vi "BCU参数读取-Auto.vi"(8 "CAN端口":u16(ring), 9 "设备索引号":u16(ring), 10 "CAN卡类型":u32(ring)=21, 11 "Myindex":dbl=1.0) -> (3 "成功":bool)   [LabVIEW 2013] (continued)
                n3273 = property on="最大允许温度" class="DigNum (严格)"("Disabled"=w5002) -> ()  [unwired: 2 in, 2 out]
                n3274 = property on="最小允许温度" class="DigNum (严格)"("Disabled"=w5002) -> ()  [unwired: 2 in, 2 out]
                n3275 = property on="最大允许充电电流" class="DigNum (严格)"("Disabled"=w5002) -> ()  [unwired: 2 in, 2 out]
                n3276 = property on="最小允许充电电流" class="DigNum (严格)"("Disabled"=w5002) -> ()  [unwired: 2 in, 2 out]
                n3277 = property on="最小允许单体电压" class="DigNum (严格)"("Disabled"=w5002) -> ()  [unwired: 2 in, 2 out]
                n3278 = property on="电流步长" class="DigNum (严格)"("Disabled"=w5002) -> ()  [unwired: 2 in, 2 out]
                n3279 = property on="SOC" class="DigNum (严格)"("Disabled"=w5002) -> ()  [unwired: 2 in, 2 out]
                n3280 = property on="充电总安时" class="DigNum (严格)"("Disabled"=w5002) -> ()  [unwired: 2 in, 2 out]
                n3281 = property on="放电总安时" class="DigNum (严格)"("Disabled"=w5002) -> ()  [unwired: 2 in, 2 out]
                n3282 = property on="放空次数" class="DigNum (严格)"("DisabledEnum"=w4994) -> ()  [unwired: 2 in, 2 out]
                n3283 = property on="充满次数" class="DigNum (严格)"("DisabledEnum"=w4994) -> ()  [unwired: 2 in, 2 out]
                n3284 = property on="充电次数" class="DigNum (严格)"("DisabledEnum"=w4994) -> ()  [unwired: 2 in, 2 out]
                n3285 = global read "功能码全局.vi" "24"() -> (w4997:bool[])
                n3286 = global read "功能码全局.vi" "23"() -> (w4998:bool[])
                n3287 = Index Array(array=w4997) -> (element #3=w4995:bool)  [unwired: 8 in, 7 out]
                n3288 = Index Array(array=w4998) -> (element #3=w4996:bool)  [unwired: 8 in, 7 out]
                n3289 = Not(x=w4991) -> (.not. x?=w5003:bool)
              }
              frame "电池包组号" {
                w5008 = 2
                w5007 = 2
                w5017 = 2
                w5009 = 2
                w5018 = 2
                w5005 = FALSE ("1 6")
                n3290 = property on="串联数" class="DigNum (严格)"("Disabled"=w5018) -> ()  [unwired: 2 in, 2 out]
                n3291 = property on="并联数" class="DigNum (严格)"("Disabled"=w5018) -> ()  [unwired: 2 in, 2 out]
                n3292 = property on="电池厂家" class="DigNum (严格)"("Disabled"=w5018) -> ()  [unwired: 2 in, 2 out]
                n3293 = property on="电池类型" class="DigNum (严格)"("Disabled"=w5018) -> ()  [unwired: 2 in, 2 out]
                n3294 = property on="额定能量" class="DigNum (严格)"("Disabled"=w5018) -> ()  [unwired: 2 in, 2 out]
                n3295 = property on="额定容量" class="DigNum (严格)"("Disabled"=w5018) -> ()  [unwired: 2 in, 2 out]
                n3296 = property on="实际容量" class="DigNum (严格)"("Disabled"=w5018) -> ()  [unwired: 2 in, 2 out]
                n3297 = Select(t=0, s=w5014, f=1) -> (s? t:f=w5006:i32)
                n3298 = property on="生产日期" class="Str"("DisabledEnum"=w5008) -> ()  [unwired: 2 in, 2 out]
                n3299 = property on="电池包序号" class="DigNum (严格)"("DisabledEnum"=w5008) -> ()  [unwired: 2 in, 2 out]
                n3300 = property on="车牌号" class="Str"("DisabledEnum"=w5008) -> ()  [unwired: 2 in, 2 out]
                n3301 = property on="电池包组号" class="DigNum (严格)"("DisabledEnum"=w5006) -> ()  [unwired: 2 in, 2 out]
                n3302 = property on="电池组信息" class="Clust (严格)"("Disabled"=w5006) -> ()  [unwired: 2 in, 2 out]
                n3303 = property on="产权标识" class="DigNum (严格)"("Disabled"=w5009) -> ()  [unwired: 2 in, 2 out]
                n3304 = property on="应用车型" class="DigNum (严格)"("Disabled"=w5009) -> ()  [unwired: 2 in, 2 out]
                n3305 = property on="额定总压" class="DigNum (严格)"("Disabled"=w5009) -> ()  [unwired: 2 in, 2 out]
                n3306 = property on="放空次数" class="DigNum (严格)"("DisabledEnum"=w5007) -> ()  [unwired: 2 in, 2 out]
                n3307 = property on="充满次数" class="DigNum (严格)"("DisabledEnum"=w5007) -> ()  [unwired: 2 in, 2 out]
                n3308 = property on="充电次数" class="DigNum (严格)"("DisabledEnum"=w5007) -> ()  [unwired: 2 in, 2 out]
                n3309 = property on="最大允许单体电压" class="DigNum (严格)"("Disabled"=w5017) -> ()  [unwired: 2 in, 2 out]
                n3310 = property on="最大允许总电压" class="DigNum (严格)"("Disabled"=w5017) -> ()  [unwired: 2 in, 2 out]
                n3311 = property on="最大允许温度" class="DigNum (严格)"("Disabled"=w5017) -> ()  [unwired: 2 in, 2 out]
                n3312 = property on="最小允许温度" class="DigNum (严格)"("Disabled"=w5017) -> ()  [unwired: 2 in, 2 out]
                n3313 = property on="最大允许充电电流" class="DigNum (严格)"("Disabled"=w5017) -> ()  [unwired: 2 in, 2 out]
                n3314 = property on="最小允许充电电流" class="DigNum (严格)"("Disabled"=w5017) -> ()  [unwired: 2 in, 2 out]
                n3315 = property on="最小允许单体电压" class="DigNum (严格)"("Disabled"=w5017) -> ()  [unwired: 2 in, 2 out]
                n3316 = property on="电流步长" class="DigNum (严格)"("Disabled"=w5017) -> ()  [unwired: 2 in, 2 out]
                n3317 = property on="SOC" class="DigNum (严格)"("Disabled"=w5017) -> ()  [unwired: 2 in, 2 out]
                n3318 = property on="充电总安时" class="DigNum (严格)"("Disabled"=w5017) -> ()  [unwired: 2 in, 2 out]
                n3319 = property on="放电总安时" class="DigNum (严格)"("Disabled"=w5017) -> ()  [unwired: 2 in, 2 out]
                n3320 = global read "功能码全局.vi" "24"() -> (w5012:bool[])
                n3321 = global read "功能码全局.vi" "23"() -> (w5013:bool[])
                n3322 = Index Array(array=w5012) -> (element #3=w5010:bool)  [unwired: 8 in, 7 out]
                n3323 = Index Array(array=w5013) -> (element #3=w5011:bool)  [unwired: 8 in, 7 out]
                n3324 = Not(x=w5005) -> (.not. x?=w5019:bool)
              }
              frame "充放电安时" {
                w5023 = 2
                w5022 = 2
                w5032 = 2
                w5033 = 2
                w5035 = 2
                w5021 = FALSE ("1 6")
                n3325 = property on="串联数" class="DigNum (严格)"("Disabled"=w5035) -> ()  [unwired: 2 in, 2 out]
                n3326 = property on="并联数" class="DigNum (严格)"("Disabled"=w5035) -> ()  [unwired: 2 in, 2 out]
                n3327 = property on="电池厂家" class="DigNum (严格)"("Disabled"=w5035) -> ()  [unwired: 2 in, 2 out]
                n3328 = property on="电池类型" class="DigNum (严格)"("Disabled"=w5035) -> ()  [unwired: 2 in, 2 out]
                n3329 = property on="额定能量" class="DigNum (严格)"("Disabled"=w5035) -> ()  [unwired: 2 in, 2 out]
                n3330 = property on="额定容量" class="DigNum (严格)"("Disabled"=w5035) -> ()  [unwired: 2 in, 2 out]
                n3331 = property on="实际容量" class="DigNum (严格)"("Disabled"=w5035) -> ()  [unwired: 2 in, 2 out]
                n3332 = Select(t=0, s=w5029, f=1) -> (s? t:f=w5028:i32)
                n3333 = property on="生产日期" class="Str"("DisabledEnum"=w5023) -> ()  [unwired: 2 in, 2 out]
                n3334 = property on="电池包序号" class="DigNum (严格)"("DisabledEnum"=w5023) -> ()  [unwired: 2 in, 2 out]
                n3335 = property on="车牌号" class="Str"("DisabledEnum"=w5023) -> ()  [unwired: 2 in, 2 out]
                n3336 = property on="电池包组号" class="DigNum (严格)"("DisabledEnum"=w5023) -> ()  [unwired: 2 in, 2 out]
                n3337 = property on="电池组信息" class="Clust (严格)"("Disabled"=w5028) -> ()  [unwired: 2 in, 2 out]
                n3338 = property on="额定总压" class="DigNum (严格)"("Disabled"=2) -> ()  [unwired: 2 in, 2 out]
                n3339 = property on="产权标识" class="DigNum (严格)"("Disabled"=w5033) -> ()  [unwired: 2 in, 2 out]
                n3340 = property on="应用车型" class="DigNum (严格)"("Disabled"=w5033) -> ()  [unwired: 2 in, 2 out]
                n3341 = property on="放空次数" class="DigNum (严格)"("DisabledEnum"=w5022) -> ()  [unwired: 2 in, 2 out]
                n3342 = property on="充满次数" class="DigNum (严格)"("DisabledEnum"=w5022) -> ()  [unwired: 2 in, 2 out]
                n3343 = property on="充电次数" class="DigNum (严格)"("DisabledEnum"=w5022) -> ()  [unwired: 2 in, 2 out]
                n3344 = property on="最大允许单体电压" class="DigNum (严格)"("Disabled"=w5032) -> ()  [unwired: 2 in, 2 out]
                n3345 = property on="最大允许总电压" class="DigNum (严格)"("Disabled"=w5032) -> ()  [unwired: 2 in, 2 out]
                n3346 = property on="最大允许温度" class="DigNum (严格)"("Disabled"=w5032) -> ()  [unwired: 2 in, 2 out]
                n3347 = property on="最小允许温度" class="DigNum (严格)"("Disabled"=w5032) -> ()  [unwired: 2 in, 2 out]
                n3348 = property on="最大允许充电电流" class="DigNum (严格)"("Disabled"=w5032) -> ()  [unwired: 2 in, 2 out]
                n3349 = property on="最小允许充电电流" class="DigNum (严格)"("Disabled"=w5032) -> ()  [unwired: 2 in, 2 out]
                n3350 = property on="最小允许单体电压" class="DigNum (严格)"("Disabled"=w5032) -> ()  [unwired: 2 in, 2 out]
                n3351 = property on="电流步长" class="DigNum (严格)"("Disabled"=w5032) -> ()  [unwired: 2 in, 2 out]
                n3352 = property on="SOC" class="DigNum (严格)"("Disabled"=w5032) -> ()  [unwired: 2 in, 2 out]
                n3353 = property on="充电总安时" class="DigNum (严格)"("Disabled"=w5028) -> ()  [unwired: 2 in, 2 out]
                n3354 = property on="放电总安时" class="DigNum (严格)"("Disabled"=w5028) -> ()  [unwired: 2 in, 2 out]
                n3355 = Not(x=w5021) -> (.not. x?=w5036:bool)
                n3356 = global read "功能码全局.vi" "24"() -> (w5026:bool[])
                n3357 = global read "功能码全局.vi" "23"() -> (w5027:bool[])
                n3358 = Index Array(array=w5026) -> (element #7=w5024:bool)  [unwired: 8 in, 7 out]
                n3359 = Index Array(array=w5027) -> (element #7=w5025:bool)  [unwired: 8 in, 7 out]
              }
              frame "充电次数" {
                w5041 = 2
                w5050 = 2
                w5051 = 2
                w5042 = 2
                w5052 = 2
                w5038 = FALSE ("1 6")
                n3360 = property on="串联数" class="DigNum (严格)"("Disabled"=w5052) -> ()  [unwired: 2 in, 2 out]
                n3361 = property on="并联数" class="DigNum (严格)"("Disabled"=w5052) -> ()  [unwired: 2 in, 2 out]
                n3362 = property on="电池厂家" class="DigNum (严格)"("Disabled"=w5052) -> ()  [unwired: 2 in, 2 out]
                n3363 = property on="电池类型" class="DigNum (严格)"("Disabled"=w5052) -> ()  [unwired: 2 in, 2 out]
                n3364 = property on="额定能量" class="DigNum (严格)"("Disabled"=w5052) -> ()  [unwired: 2 in, 2 out]
                n3365 = property on="额定容量" class="DigNum (严格)"("Disabled"=w5052) -> ()  [unwired: 2 in, 2 out]
                n3366 = property on="实际容量" class="DigNum (严格)"("Disabled"=w5052) -> ()  [unwired: 2 in, 2 out]
                n3367 = Select(t=0, s=w5047, f=1) -> (s? t:f=w5039:i32)
                n3368 = property on="生产日期" class="Str"("DisabledEnum"=w5041) -> ()  [unwired: 2 in, 2 out]
                n3369 = property on="电池包序号" class="DigNum (严格)"("DisabledEnum"=w5041) -> ()  [unwired: 2 in, 2 out]
                n3370 = property on="车牌号" class="Str"("DisabledEnum"=w5041) -> ()  [unwired: 2 in, 2 out]
                n3371 = property on="电池组信息" class="Clust (严格)"("Disabled"=w5039) -> ()  [unwired: 2 in, 2 out]
                n3372 = property on="电池包组号" class="DigNum (严格)"("DisabledEnum"=w5041) -> ()  [unwired: 2 in, 2 out]
                n3373 = property on="额定总压" class="DigNum (严格)"("Disabled"=w5042) -> ()  [unwired: 2 in, 2 out]
                n3374 = property on="产权标识" class="DigNum (严格)"("Disabled"=w5042) -> ()  [unwired: 2 in, 2 out]
                n3375 = property on="应用车型" class="DigNum (严格)"("Disabled"=w5042) -> ()  [unwired: 2 in, 2 out]
                n3376 = property on="放空次数" class="DigNum (严格)"("DisabledEnum"=w5039) -> (error out=w5040:errorcluster)  [unwired: 2 in, 1 out]
                n3377 = property on="充满次数" class="DigNum (严格)"("DisabledEnum"=w5039) -> ()  [unwired: 2 in, 2 out]
                n3378 = property on="充电次数" class="DigNum (严格)"("DisabledEnum"=w5039) -> ()  [unwired: 2 in, 2 out]
                n3379 = property on="最大允许单体电压" class="DigNum (严格)"("Disabled"=w5051) -> ()  [unwired: 2 in, 2 out]
                n3380 = property on="最大允许总电压" class="DigNum (严格)"("Disabled"=w5051) -> ()  [unwired: 2 in, 2 out]
                n3381 = property on="最大允许温度" class="DigNum (严格)"("Disabled"=w5051) -> ()  [unwired: 2 in, 2 out]
                n3382 = property on="最小允许温度" class="DigNum (严格)"("Disabled"=w5051) -> ()  [unwired: 2 in, 2 out]
                n3383 = property on="最大允许充电电流" class="DigNum (严格)"("Disabled"=w5051) -> ()  [unwired: 2 in, 2 out]
                n3384 = property on="最小允许充电电流" class="DigNum (严格)"(error in=w5040, "Disabled"=w5051) -> ()  [unwired: 1 in, 2 out]
                n3385 = property on="最小允许单体电压" class="DigNum (严格)"("Disabled"=w5051) -> ()  [unwired: 2 in, 2 out]
                n3386 = property on="电流步长" class="DigNum (严格)"("Disabled"=w5051) -> ()  [unwired: 2 in, 2 out]
                n3387 = property on="SOC" class="DigNum (严格)"("Disabled"=w5051) -> ()  [unwired: 2 in, 2 out]
                n3388 = property on="充电总安时" class="DigNum (严格)"("Disabled"=w5050) -> ()  [unwired: 2 in, 2 out]
                n3389 = property on="放电总安时" class="DigNum (严格)"("Disabled"=w5050) -> ()  [unwired: 2 in, 2 out]
                n3390 = Not(x=w5038) -> (.not. x?=w5053:bool)
                n3391 = global read "功能码全局.vi" "24"() -> (w5045:bool[])
                n3392 = global read "功能码全局.vi" "23"() -> (w5046:bool[])
                n3393 = Index Array(array=w5045) -> (element #8=w5044:bool)  [unwired: 8 in, 7 out]
                n3394 = Index Array(array=w5046) -> (element #8=w5043:bool)  [unwired: 8 in, 7 out]
              }
              frame "SOC" {
                w5057 = 2
                w5056 = 2
                w5066 = 2
                w5067 = 2
                w5068 = 2
                w5070 = 2
                w5055 = FALSE ("1 6")
                n3395 = property on="串联数" class="DigNum (严格)"("Disabled"=w5070) -> ()  [unwired: 2 in, 2 out]
                n3396 = property on="并联数" class="DigNum (严格)"("Disabled"=w5070) -> ()  [unwired: 2 in, 2 out]
                n3397 = property on="电池厂家" class="DigNum (严格)"("Disabled"=w5070) -> ()  [unwired: 2 in, 2 out]
                n3398 = property on="电池类型" class="DigNum (严格)"("Disabled"=w5070) -> ()  [unwired: 2 in, 2 out]
                n3399 = property on="额定能量" class="DigNum (严格)"("Disabled"=w5070) -> ()  [unwired: 2 in, 2 out]
                n3400 = property on="额定容量" class="DigNum (严格)"("Disabled"=w5070) -> ()  [unwired: 2 in, 2 out]
                n3401 = property on="实际容量" class="DigNum (严格)"("Disabled"=w5070) -> ()  [unwired: 2 in, 2 out]
                n3402 = Select(t=0, s=w5063, f=1) -> (s? t:f=w5062:i32)
                n3403 = property on="生产日期" class="Str"("DisabledEnum"=w5057) -> ()  [unwired: 2 in, 2 out]
                n3404 = property on="电池包序号" class="DigNum (严格)"("DisabledEnum"=w5057) -> ()  [unwired: 2 in, 2 out]
                n3405 = property on="车牌号" class="Str"("DisabledEnum"=w5057) -> ()  [unwired: 2 in, 2 out]
                n3406 = property on="电池包组号" class="DigNum (严格)"("DisabledEnum"=w5057) -> ()  [unwired: 2 in, 2 out]
                n3407 = property on="电池组信息" class="Clust (严格)"("Disabled"=w5062) -> ()  [unwired: 2 in, 2 out]
                n3408 = property on="SOC" class="DigNum (严格)"("Disabled"=w5062) -> ()  [unwired: 2 in, 2 out]
                n3409 = property on="额定总压" class="DigNum (严格)"("Disabled"=2) -> ()  [unwired: 2 in, 2 out]
                n3410 = property on="产权标识" class="DigNum (严格)"("Disabled"=w5068) -> ()  [unwired: 2 in, 2 out]
                n3411 = property on="应用车型" class="DigNum (严格)"("Disabled"=w5068) -> ()  [unwired: 2 in, 2 out]
                n3412 = property on="放空次数" class="DigNum (严格)"("DisabledEnum"=w5056) -> ()  [unwired: 2 in, 2 out]
                n3413 = property on="充满次数" class="DigNum (严格)"("DisabledEnum"=w5056) -> ()  [unwired: 2 in, 2 out]
                n3414 = property on="充电次数" class="DigNum (严格)"("DisabledEnum"=w5056) -> ()  [unwired: 2 in, 2 out]
                n3415 = property on="最大允许单体电压" class="DigNum (严格)"("Disabled"=w5067) -> ()  [unwired: 2 in, 2 out]
                n3416 = property on="最大允许总电压" class="DigNum (严格)"("Disabled"=w5067) -> ()  [unwired: 2 in, 2 out]
                n3417 = property on="最大允许温度" class="DigNum (严格)"("Disabled"=w5067) -> ()  [unwired: 2 in, 2 out]
                n3418 = property on="最小允许温度" class="DigNum (严格)"("Disabled"=w5067) -> ()  [unwired: 2 in, 2 out]
                n3419 = property on="最大允许充电电流" class="DigNum (严格)"("Disabled"=w5067) -> ()  [unwired: 2 in, 2 out]
                n3420 = property on="最小允许充电电流" class="DigNum (严格)"("Disabled"=w5067) -> ()  [unwired: 2 in, 2 out]
                n3421 = property on="最小允许单体电压" class="DigNum (严格)"("Disabled"=w5067) -> ()  [unwired: 2 in, 2 out]
                n3422 = property on="电流步长" class="DigNum (严格)"("Disabled"=w5067) -> ()  [unwired: 2 in, 2 out]
                n3423 = property on="充电总安时" class="DigNum (严格)"("Disabled"=w5066) -> ()  [unwired: 2 in, 2 out]
                n3424 = property on="放电总安时" class="DigNum (严格)"("Disabled"=w5066) -> ()  [unwired: 2 in, 2 out]
                n3425 = Not(x=w5055) -> (.not. x?=w5071:bool)
                n3426 = global read "功能码全局.vi" "24"() -> (w5060:bool[])
                n3427 = global read "功能码全局.vi" "23"() -> (w5061:bool[])
                n3428 = Index Array(array=w5060) -> (element #6=w5059:bool)  [unwired: 8 in, 7 out]
                n3429 = Index Array(array=w5061) -> (element #6=w5058:bool)  [unwired: 8 in, 7 out]
              }
              frame "车牌号" {
                w5076 = 2
                w5075 = 2
                w5085 = 2
                w5086 = 2
                w5087 = 2
                w5089 = 2
                w5073 = FALSE ("1 6")
                n3430 = property on="串联数" class="DigNum (严格)"("Disabled"=w5089) -> ()  [unwired: 2 in, 2 out]
                n3431 = property on="并联数" class="DigNum (严格)"("Disabled"=w5089) -> ()  [unwired: 2 in, 2 out]
                n3432 = property on="电池厂家" class="DigNum (严格)"("Disabled"=w5089) -> ()  [unwired: 2 in, 2 out]
                n3433 = property on="电池类型" class="DigNum (严格)"("Disabled"=w5089) -> ()  [unwired: 2 in, 2 out]
                n3434 = property on="额定能量" class="DigNum (严格)"("Disabled"=w5089) -> ()  [unwired: 2 in, 2 out]
                n3435 = property on="额定容量" class="DigNum (严格)"("Disabled"=w5089) -> ()  [unwired: 2 in, 2 out]
                n3436 = property on="实际容量" class="DigNum (严格)"("Disabled"=w5089) -> ()  [unwired: 2 in, 2 out]
                n3437 = Select(t=0, s=w5081, f=1) -> (s? t:f=w5074:i32)
                n3438 = property on="生产日期" class="Str"("DisabledEnum"=w5076) -> ()  [unwired: 2 in, 2 out]
                n3439 = property on="电池包序号" class="DigNum (严格)"("DisabledEnum"=w5076) -> ()  [unwired: 2 in, 2 out]
                n3440 = property on="电池包组号" class="DigNum (严格)"("DisabledEnum"=w5076) -> ()  [unwired: 2 in, 2 out]
                n3441 = property on="电池组信息" class="Clust (严格)"("Disabled"=w5074) -> ()  [unwired: 2 in, 2 out]
                n3442 = property on="车牌号" class="Str"("DisabledEnum"=w5074) -> ()  [unwired: 2 in, 2 out]
                n3443 = property on="额定总压" class="DigNum (严格)"("Disabled"=2) -> ()  [unwired: 2 in, 2 out]
                n3444 = property on="产权标识" class="DigNum (严格)"("Disabled"=w5087) -> ()  [unwired: 2 in, 2 out]
                n3445 = property on="应用车型" class="DigNum (严格)"("Disabled"=w5087) -> ()  [unwired: 2 in, 2 out]
                n3446 = property on="放空次数" class="DigNum (严格)"("DisabledEnum"=w5075) -> ()  [unwired: 2 in, 2 out]
                n3447 = property on="充满次数" class="DigNum (严格)"("DisabledEnum"=w5075) -> ()  [unwired: 2 in, 2 out]
                n3448 = property on="充电次数" class="DigNum (严格)"("DisabledEnum"=w5075) -> ()  [unwired: 2 in, 2 out]
                n3449 = property on="最大允许单体电压" class="DigNum (严格)"("Disabled"=w5086) -> ()  [unwired: 2 in, 2 out]
                n3450 = property on="最大允许总电压" class="DigNum (严格)"("Disabled"=w5086) -> ()  [unwired: 2 in, 2 out]
                n3451 = property on="最大允许温度" class="DigNum (严格)"("Disabled"=w5086) -> ()  [unwired: 2 in, 2 out]
                n3452 = property on="最小允许温度" class="DigNum (严格)"("Disabled"=w5086) -> ()  [unwired: 2 in, 2 out]
                n3453 = property on="最大允许充电电流" class="DigNum (严格)"("Disabled"=w5086) -> ()  [unwired: 2 in, 2 out]
                n3454 = property on="最小允许充电电流" class="DigNum (严格)"("Disabled"=w5086) -> ()  [unwired: 2 in, 2 out]
                n3455 = property on="最小允许单体电压" class="DigNum (严格)"("Disabled"=w5086) -> ()  [unwired: 2 in, 2 out]
                n3456 = property on="电流步长" class="DigNum (严格)"("Disabled"=w5086) -> ()  [unwired: 2 in, 2 out]
                n3457 = property on="SOC" class="DigNum (严格)"("Disabled"=2) -> ()  [unwired: 2 in, 2 out]
                n3458 = property on="充电总安时" class="DigNum (严格)"("Disabled"=w5085) -> ()  [unwired: 2 in, 2 out]
                n3459 = property on="放电总安时" class="DigNum (严格)"("Disabled"=w5085) -> ()  [unwired: 2 in, 2 out]
                n3460 = Not(x=w5073) -> (.not. x?=w5090:bool)
                n3461 = global read "功能码全局.vi" "24"() -> (w5079:bool[])
                n3462 = global read "功能码全局.vi" "23"() -> (w5080:bool[])
                n3463 = Index Array(array=w5079) -> (element #5=w5077:bool)  [unwired: 8 in, 7 out]
                n3464 = Index Array(array=w5080) -> (element #5=w5078:bool)  [unwired: 8 in, 7 out]
              }
              frame "充电参数" {
                w5094 = 2
                w5093 = 2
                w5103 = 2
                w5104 = 2
                w5106 = 2
                w5092 = FALSE ("1 6")
                n3465 = property on="串联数" class="DigNum (严格)"("Disabled"=w5106) -> ()  [unwired: 2 in, 2 out]
                n3466 = property on="并联数" class="DigNum (严格)"("Disabled"=w5106) -> ()  [unwired: 2 in, 2 out]
                n3467 = property on="电池厂家" class="DigNum (严格)"("Disabled"=w5106) -> ()  [unwired: 2 in, 2 out]
                n3468 = property on="电池类型" class="DigNum (严格)"("Disabled"=w5106) -> ()  [unwired: 2 in, 2 out]
                n3469 = property on="额定能量" class="DigNum (严格)"("Disabled"=w5106) -> ()  [unwired: 2 in, 2 out]
                n3470 = property on="额定容量" class="DigNum (严格)"("Disabled"=w5106) -> ()  [unwired: 2 in, 2 out]
                n3471 = property on="实际容量" class="DigNum (严格)"("Disabled"=w5106) -> ()  [unwired: 2 in, 2 out]
                n3472 = Select(t=0, s=w5100, f=1) -> (s? t:f=w5099:i32)
                n3473 = property on="生产日期" class="Str"("DisabledEnum"=w5094) -> ()  [unwired: 2 in, 2 out]
                n3474 = property on="电池包序号" class="DigNum (严格)"("DisabledEnum"=w5094) -> ()  [unwired: 2 in, 2 out]
                n3475 = property on="车牌号" class="Str"("DisabledEnum"=w5094) -> ()  [unwired: 2 in, 2 out]
                n3476 = property on="电池组信息" class="Clust (严格)"("Disabled"=w5099) -> ()  [unwired: 2 in, 2 out]
                n3477 = property on="电池包组号" class="DigNum (严格)"("DisabledEnum"=w5094) -> ()  [unwired: 2 in, 2 out]
                n3478 = property on="额定总压" class="DigNum (严格)"("Disabled"=2) -> ()  [unwired: 2 in, 2 out]
                n3479 = property on="产权标识" class="DigNum (严格)"("Disabled"=w5104) -> ()  [unwired: 2 in, 2 out]
                n3480 = property on="应用车型" class="DigNum (严格)"("Disabled"=w5104) -> ()  [unwired: 2 in, 2 out]
                n3481 = property on="放空次数" class="DigNum (严格)"("DisabledEnum"=w5093) -> ()  [unwired: 2 in, 2 out]
                n3482 = property on="充满次数" class="DigNum (严格)"("DisabledEnum"=w5093) -> ()  [unwired: 2 in, 2 out]
                n3483 = property on="充电次数" class="DigNum (严格)"("DisabledEnum"=w5093) -> ()  [unwired: 2 in, 2 out]
                n3484 = property on="最大允许单体电压" class="DigNum (严格)"("Disabled"=w5099) -> ()  [unwired: 2 in, 2 out]
                n3485 = property on="最大允许总电压" class="DigNum (严格)"("Disabled"=w5099) -> ()  [unwired: 2 in, 2 out]
                n3486 = property on="最大允许温度" class="DigNum (严格)"("Disabled"=w5099) -> ()  [unwired: 2 in, 2 out]
                n3487 = property on="最小允许温度" class="DigNum (严格)"("Disabled"=w5099) -> ()  [unwired: 2 in, 2 out]
                n3488 = property on="最大允许充电电流" class="DigNum (严格)"("Disabled"=w5099) -> ()  [unwired: 2 in, 2 out]
                n3489 = property on="最小允许充电电流" class="DigNum (严格)"("Disabled"=w5099) -> ()  [unwired: 2 in, 2 out]
                n3490 = property on="最小允许单体电压" class="DigNum (严格)"("Disabled"=w5099) -> ()  [unwired: 2 in, 2 out]
                n3491 = property on="电流步长" class="DigNum (严格)"("Disabled"=w5099) -> ()  [unwired: 2 in, 2 out]
                n3492 = property on="SOC" class="DigNum (严格)"("Disabled"=w5103) -> ()  [unwired: 2 in, 2 out]
                n3493 = property on="充电总安时" class="DigNum (严格)"("Disabled"=w5103) -> ()  [unwired: 2 in, 2 out]
                n3494 = property on="放电总安时" class="DigNum (严格)"("Disabled"=w5103) -> ()  [unwired: 2 in, 2 out]
                n3495 = Not(x=w5092) -> (.not. x?=w5107:bool)
                n3496 = global read "功能码全局.vi" "24"() -> (w5097:bool[])
                n3497 = global read "功能码全局.vi" "23"() -> (w5098:bool[])
                n3498 = Index Array(array=w5097) -> (element #4=w5095:bool)  [unwired: 8 in, 7 out]
                n3499 = Index Array(array=w5098) -> (element #4=w5096:bool)  [unwired: 8 in, 7 out]
              }
              frame "均衡参数" {
                w5109 = FALSE ("1 6")
                n3500 = Select(t=0, s=w5115, f=1) -> (s? t:f=w5113:i32)
                n3501 = property on="均衡计算-电压高阀值1级" class="DigNum (严格)"("DisabledEnum"=w5113) -> ()  [unwired: 2 in, 2 out]
                n3502 = property on="均衡计算-电压高阀值2级" class="DigNum (严格)"("DisabledEnum"=w5113) -> ()  [unwired: 2 in, 2 out]
                n3503 = property on="均衡计算-电压低阀值1级" class="DigNum (严格)"("DisabledEnum"=w5113) -> ()  [unwired: 2 in, 2 out]
                n3504 = property on="均衡计算-电压低阀值2级" class="DigNum (严格)"("DisabledEnum"=w5113) -> ()  [unwired: 2 in, 2 out]
                n3505 = property on="均衡计算-最低电压阀值" class="DigNum (严格)"("DisabledEnum"=w5113) -> ()  [unwired: 2 in, 2 out]
                n3506 = property on="均衡停止-最低电压阀值" class="DigNum (严格)"("DisabledEnum"=w5113) -> ()  [unwired: 2 in, 2 out]
                n3507 = property on="均衡计算-电压极差阀值" class="DigNum (严格)"("DisabledEnum"=w5113) -> ()  [unwired: 2 in, 2 out]
                n3508 = property on="均衡参数" class="Clust (严格)"("DisabledEnum"=w5113) -> ()  [unwired: 2 in, 2 out]
                n3509 = property on="充电结束电压(90%)" class="DigNum (严格)"("DisabledEnum"=w5113) -> ()  [unwired: 2 in, 2 out]
                n3510 = property on="充电结束电压(91%)" class="DigNum (严格)"("DisabledEnum"=w5113) -> ()  [unwired: 2 in, 2 out]
                n3511 = property on="充电结束电压(92%)" class="DigNum (严格)"("DisabledEnum"=w5113) -> ()  [unwired: 2 in, 2 out]
                n3512 = property on="充电结束电压(93%)" class="DigNum (严格)"("DisabledEnum"=w5113) -> ()  [unwired: 2 in, 2 out]
                n3513 = property on="充电结束电压(94%)" class="DigNum (严格)"("DisabledEnum"=w5113) -> ()  [unwired: 2 in, 2 out]
                n3514 = property on="充电结束电压(95%)" class="DigNum (严格)"("DisabledEnum"=w5113) -> ()  [unwired: 2 in, 2 out]
                n3515 = property on="充电结束电压(96%)" class="DigNum (严格)"("DisabledEnum"=w5113) -> ()  [unwired: 2 in, 2 out]
                n3516 = property on="充电结束电压(97%)" class="DigNum (严格)"("DisabledEnum"=w5113) -> ()  [unwired: 2 in, 2 out]
                n3517 = property on="充电结束电压(98%)" class="DigNum (严格)"("DisabledEnum"=w5113) -> ()  [unwired: 2 in, 2 out]
                n3518 = property on="充电结束电压(99%)" class="DigNum (严格)"("DisabledEnum"=w5113) -> ()  [unwired: 2 in, 2 out]
                n3519 = property on="充电结束电压(100%)" class="DigNum (严格)"("DisabledEnum"=w5113) -> ()  [unwired: 2 in, 2 out]
                n3520 = disable-structure shown="启用" {
                  disable-tunnel: [w5119 w5121] -> w5112
                  disable-tunnel: [w5118 w5121] -> w5111
                  frame Enabled {
                    n3521 = global read "功能码全局.vi" "18"() -> (w5120:bool[])
                    n3522 = Index Array(array=w5120) -> (element #1=w5119:bool, element #2=w5118:bool)  [unwired: 8 in, 6 out]
                  }
                  frame Disabled {
                    w5121 = TRUE
                  }
                }
                n3523 = Not(x=w5109) -> (.not. x?=w5110:bool)
              }
              frame "均衡阀值" {
                w5124 = 2
                w5122 = FALSE ("1 6")
                n3524 = Select(t=0, s=w5129, f=1) -> (s? t:f=w5127:i32)
                n3525 = property on="均衡计算-电压高阀值1级" class="DigNum (严格)"("DisabledEnum"=w5127) -> ()  [unwired: 2 in, 2 out]
                n3526 = property on="均衡计算-电压高阀值2级" class="DigNum (严格)"("DisabledEnum"=w5127) -> ()  [unwired: 2 in, 2 out]
                n3527 = property on="均衡计算-电压低阀值1级" class="DigNum (严格)"("DisabledEnum"=w5127) -> ()  [unwired: 2 in, 2 out]
                n3528 = property on="均衡计算-电压低阀值2级" class="DigNum (严格)"("DisabledEnum"=w5127) -> ()  [unwired: 2 in, 2 out]
                n3529 = property on="均衡计算-最低电压阀值" class="DigNum (严格)"("DisabledEnum"=w5127) -> ()  [unwired: 2 in, 2 out]
                n3530 = property on="均衡停止-最低电压阀值" class="DigNum (严格)"("DisabledEnum"=w5127) -> ()  [unwired: 2 in, 2 out]
                n3531 = property on="均衡计算-电压极差阀值" class="DigNum (严格)"("DisabledEnum"=w5127) -> ()  [unwired: 2 in, 2 out]
                n3532 = property on="均衡参数" class="Clust (严格)"("DisabledEnum"=w5127) -> ()  [unwired: 2 in, 2 out]
                n3533 = property on="充电结束电压(90%)" class="DigNum (严格)"("DisabledEnum"=w5124) -> ()  [unwired: 2 in, 2 out]
                n3534 = property on="充电结束电压(91%)" class="DigNum (严格)"("DisabledEnum"=w5124) -> ()  [unwired: 2 in, 2 out]
                n3535 = property on="充电结束电压(92%)" class="DigNum (严格)"("DisabledEnum"=w5124) -> ()  [unwired: 2 in, 2 out]
                n3536 = property on="充电结束电压(93%)" class="DigNum (严格)"("DisabledEnum"=w5124) -> ()  [unwired: 2 in, 2 out]
                n3537 = property on="充电结束电压(94%)" class="DigNum (严格)"("DisabledEnum"=w5124) -> ()  [unwired: 2 in, 2 out]
                n3538 = property on="充电结束电压(95%)" class="DigNum (严格)"("DisabledEnum"=w5124) -> ()  [unwired: 2 in, 2 out]
                n3539 = property on="充电结束电压(96%)" class="DigNum (严格)"("DisabledEnum"=w5124) -> ()  [unwired: 2 in, 2 out]
                n3540 = property on="充电结束电压(97%)" class="DigNum (严格)"("DisabledEnum"=w5124) -> ()  [unwired: 2 in, 2 out]
                n3541 = property on="充电结束电压(98%)" class="DigNum (严格)"("DisabledEnum"=w5124) -> ()  [unwired: 2 in, 2 out]
                n3542 = property on="充电结束电压(99%)" class="DigNum (严格)"("DisabledEnum"=w5124) -> ()  [unwired: 2 in, 2 out]
                n3543 = property on="充电结束电压(100%)" class="DigNum (严格)"("DisabledEnum"=w5124) -> ()  [unwired: 2 in, 2 out]
                n3544 = disable-structure shown="启用" {
                  disable-tunnel: [w5133 w5135] -> w5126
                  disable-tunnel: [w5132 w5135] -> w5125
                  frame Enabled {
                    n3545 = global read "功能码全局.vi" "18"() -> (w5134:bool[])
                    n3546 = Index Array(array=w5134) -> (element #1=w5133:bool, element #2=w5132:bool)  [unwired: 8 in, 6 out]
                  }
                  frame Disabled {
                    w5135 = TRUE
                  }
                }
                n3547 = Not(x=w5122) -> (.not. x?=w5123:bool)
              }
              frame "充电结束电压" {
                w5139 = 2
                w5136 = FALSE ("1 6")
                n3548 = Select(t=0, s=w5143, f=1) -> (s? t:f=w5138:i32)
                n3549 = property on="均衡计算-电压高阀值1级" class="DigNum (严格)"("DisabledEnum"=w5139) -> ()  [unwired: 2 in, 2 out]
                n3550 = property on="均衡计算-电压高阀值2级" class="DigNum (严格)"("DisabledEnum"=w5139) -> ()  [unwired: 2 in, 2 out]
                n3551 = property on="均衡计算-电压低阀值1级" class="DigNum (严格)"("DisabledEnum"=w5139) -> ()  [unwired: 2 in, 2 out]
                n3552 = property on="均衡计算-电压低阀值2级" class="DigNum (严格)"("DisabledEnum"=w5139) -> ()  [unwired: 2 in, 2 out]
                n3553 = property on="均衡计算-最低电压阀值" class="DigNum (严格)"("DisabledEnum"=w5139) -> ()  [unwired: 2 in, 2 out]
                n3554 = property on="均衡停止-最低电压阀值" class="DigNum (严格)"("DisabledEnum"=w5139) -> ()  [unwired: 2 in, 2 out]
                n3555 = property on="均衡计算-电压极差阀值" class="DigNum (严格)"("DisabledEnum"=w5139) -> ()  [unwired: 2 in, 2 out]
                n3556 = property on="均衡参数" class="Clust (严格)"("DisabledEnum"=w5138) -> ()  [unwired: 2 in, 2 out]
                n3557 = property on="充电结束电压(90%)" class="DigNum (严格)"("DisabledEnum"=w5138) -> ()  [unwired: 2 in, 2 out]
                n3558 = property on="充电结束电压(91%)" class="DigNum (严格)"("DisabledEnum"=w5138) -> ()  [unwired: 2 in, 2 out]
                n3559 = property on="充电结束电压(92%)" class="DigNum (严格)"("DisabledEnum"=w5138) -> ()  [unwired: 2 in, 2 out]
                n3560 = property on="充电结束电压(93%)" class="DigNum (严格)"("DisabledEnum"=w5138) -> ()  [unwired: 2 in, 2 out]
                n3561 = property on="充电结束电压(94%)" class="DigNum (严格)"("DisabledEnum"=w5138) -> ()  [unwired: 2 in, 2 out]
                n3562 = property on="充电结束电压(95%)" class="DigNum (严格)"("DisabledEnum"=w5138) -> ()  [unwired: 2 in, 2 out]
                n3563 = property on="充电结束电压(96%)" class="DigNum (严格)"("DisabledEnum"=w5138) -> ()  [unwired: 2 in, 2 out]
                n3564 = property on="充电结束电压(97%)" class="DigNum (严格)"("DisabledEnum"=w5138) -> ()  [unwired: 2 in, 2 out]
                n3565 = property on="充电结束电压(98%)" class="DigNum (严格)"("DisabledEnum"=w5138) -> ()  [unwired: 2 in, 2 out]
                n3566 = property on="充电结束电压(99%)" class="DigNum (严格)"("DisabledEnum"=w5138) -> ()  [unwired: 2 in, 2 out]
                n3567 = property on="充电结束电压(100%)" class="DigNum (严格)"("DisabledEnum"=w5138) -> ()  [unwired: 2 in, 2 out]
                n3568 = disable-structure shown="启用" {
                  disable-tunnel: [w5147 w5149] -> w5141
                  disable-tunnel: [w5146 w5149] -> w5140
                  frame Enabled {
                    n3569 = global read "功能码全局.vi" "18"() -> (w5148:bool[])
                    n3570 = Index Array(array=w5148) -> (element #1=w5147:bool, element #2=w5146:bool)  [unwired: 8 in, 6 out]
                  }
                  frame Disabled {
                    w5149 = TRUE
                  }
                }
                n3571 = Not(x=w5136) -> (.not. x?=w5137:bool)
              }
              frame "假", Default {
                w5150 = FALSE ("1 6")
                n3572 = Not(x=w5150) -> (.not. x?=w5151:bool)
              }
            }
            n3573 = local write "等级 2"(w4731) -> ()
            n3574 = local write "1 6"(w4730) -> ()
            n3575 = local write "1 7"(w4729) -> ()
            n3576 = local write "1 8"(w4728) -> ()
            n3577 = local write "1 9"(w4727) -> ()
            n3578 = local write "1 10"(w4726) -> ()
            n3579 = local write "1 12"(w4720) -> ()
            n3580 = property on="单个读取" class="Bool (严格)"("Visible"=w4725) -> ()  [unwired: 2 in, 2 out]
            n3581 = property on="单个写入" class="Bool (严格)"("Visible"=w4724) -> ()  [unwired: 2 in, 2 out]
          }
          event "从板个数": Value Change {
            n3582 = event-data() -> ()  [unwired: 7 out]
            n3583 = local read "从板个数"() -> (w5153:dbl)
            n3584 = call "多从板对应参数-new.vi"("从板个数"=w5153) -> ("输出数组"=w5154:string[])  [unwired: 1 in]
            n3585 = control-ref of="项目信息"() -> (w5155:refnum<vi>)
            n3586 = stacked-sequence {
              tunnel: w5155 -> [_ w5162 w5166]
              tunnel: w5154 -> [_ w5161 w5165]
              frame #0 {
                n3587 = local write "项目信息"(string[][] [] ("项目信息")) -> ()
              }
              frame #1 {
                n3588 = call "表格数据输入-8.6.vi"("行数"=u32 0, "列数"=u32 0, "字符串数组"=w5161, "表格引用"=w5162) -> ()  [unwired: 8 out]
              }
              frame #2 {
                n3589 = Array Size(array=w5165) -> (size(s)=w5164:i32)
                n3590 = for {
                  N: w5164 -> [_]
                  tunnel: [""] -> w5163 mode=indexing
                }
                n3591 = call "表格数据输入-8.6.vi"("行数"=u32 0, "列数"=u32 1, "字符串数组"=w5163, "表格引用"=w5166) -> ()  [unwired: 8 out]
              }
            }
          }
          event "主界面选项": Value Change {
            n3592 = event-data() -> ("NewVal"=w5170:enum32{"单选选项1", "单选选项2", "单选选项2 2", "单选选项2 3"})  [unwired: 6 out]
            n3593 = control-ref of="单选选项2 2"() -> (w5175:refnum<vi>)
            n3594 = control-ref of="单选选项2"() -> (w5177:refnum<vi>)
            n3595 = control-ref of="单选选项1"() -> (w5176:refnum<vi>)
            n3596 = control-ref of="单选选项2 3"() -> (w5171:refnum<vi>)
            n3597 = Build Array(w5176, w5177, w5175, w5171) -> (w5174:refnum<vi>[])
            n3598 = case shown="\"单选选项2 2\"" w5170 {
              selector: w5170 -> [w5188 w5193 w5198 w5203]
              tunnel: w5174 -> [w5189 w5194 w5199 w5204]
              tunnel: [w5187 w5192 w5197 w5202] -> w5180
              tunnel: [w5186 w5191 w5196 w5201] -> w5179
              tunnel: [enum32{"读写参数", "版本读取", "其它诊断"}."读写参数" ("选项卡控件 2") enum32{"读写参数", "版本读取", "其它诊断"}."版本读取" ("选项卡控件 2") enum32{"读写参数", "版本读取", "其它诊断"}."其它诊断" ("选项卡控件 2") enum32{"读写参数", "版本读取", "其它诊断", "高压板校正"}."高压板校正" ("选项卡控件 2")] -> w5178
              frame "单选选项1", Default {
                n3599 = Delete From Array(array=w5189, index=w5188) -> (deleted portion=w5186:refnum<vi>, array with subset deleted=w5187:refnum<vi>[])  [unwired: 1 in]
              }
              frame "单选选项2" {
                n3600 = Delete From Array(array=w5194, index=w5193) -> (deleted portion=w5191:refnum<vi>, array with subset deleted=w5192:refnum<vi>[])  [unwired: 1 in]
              }
              frame "单选选项2 2" {
                n3601 = Delete From Array(array=w5199, index=w5198) -> (deleted portion=w5196:refnum<vi>, array with subset deleted=w5197:refnum<vi>[])  [unwired: 1 in]
              }
              frame "单选选项2 3" {
                n3602 = Delete From Array(array=w5204, index=w5203) -> (deleted portion=w5201:refnum<vi>, array with subset deleted=w5202:refnum<vi>[])  [unwired: 1 in]
              }
            }
            n3603 = local write "面板选择"(w5178) -> ()
            n3604 = for {
              tunnel: u32 16777215 -> [w5184]
              tunnel: w5180 -> [w5183] mode=indexing
              n3605 = property class="Bool (严格)"(reference=w5183, "BoolText.TextColor"=w5184) -> ()  [unwired: 1 in, 2 out]
            }
            n3606 = property class="Bool (严格)"(reference=w5179, "BoolText.TextColor"=u32 65511) -> ()  [unwired: 1 in, 2 out]
          }
          event "主从板": Value Change {
            w5206 = FALSE ("可见")
            n3607 = event-data() -> ()  [unwired: 7 out]
            n3608 = control-ref of="单选选项2"() -> (w5214:refnum<vi>)
            n3609 = control-ref of="单选选项1"() -> (w5213:refnum<vi>)
            n3610 = local read "主从板"() -> (w5221:enum32{"单选选项2", "单选选项1"})
            n3611 = Build Array(w5214, w5213) -> (w5220:refnum<vi>[])
            n3612 = case shown="\"单选选项2\"" w5221 {
              selector: w5221 -> [w5266 w5309]
              tunnel: w5220 -> [w5267 w5308]
              tunnel: [enum32{"主板", "从板"}."主板" ("主从选择") enum32{"主板", "从板"}."从板" ("主从选择")] -> w5219
              tunnel: [w5265 w5307] -> w5216
              tunnel: [w5264 w5306] -> w5215
              tunnel: [TRUE FALSE] -> w5211
              tunnel: [w5225 w5286] -> w5208
              tunnel: [w5226 w5291] -> w5207
              tunnel: [FALSE ("可见") TRUE ("可见")] -> w5205
              frame "单选选项1", Default {
                n3613 = global read "功能码全局.vi" "主板项目信息7"() -> (w5237:bool[])
                n3614 = global read "功能码全局.vi" "主板项目信息4"() -> (w5260:bool[])
                n3615 = global read "功能码全局.vi" "主板控制类信息10"() -> (w5241:bool[])
                n3616 = global read "功能码全局.vi" "主板故障阀值9"() -> (w5238:bool[])
                n3617 = global read "功能码全局.vi" "主板项目信息5"() -> (w5251:bool[])
                n3618 = global read "功能码全局.vi" "主板项目信息6"() -> (w5261:bool[])
                n3619 = global read "功能码全局.vi" "主板版本号11"() -> (w5252:bool[])
                n3620 = Delete From Array(array=w5261, length=1 ("长度"), index=0 ("索引")) -> (deleted portion=w5250:bool[], array with subset deleted=w5233:bool[])
                n3621 = Index Array(array=w5260, index #1=5 ("索引"), index #2=6 ("索引")) -> (element #1=w5249:bool, element #2=w5232:bool)
                n3622 = Index Array(array=w5252) -> (element #1=w5245:bool, element #2=w5228:bool)  [unwired: 2 in]
                n3623 = Array Subset(array=w5238, index=2 ("索引"), length=3 ("长度")) -> (w5247:bool[])
                n3624 = Delete From Array(array=w5237, length=3 ("索引"), index=2 ("长度")) -> (deleted portion=w5248:bool[], array with subset deleted=w5231:bool[])
                n3625 = Array Subset(array=w5241, index=4 ("索引"), length=2 ("长度")) -> (w5246:bool[])
                n3626 = Delete From Array(array=w5267, index=w5266) -> (deleted portion=w5264:refnum<vi>, array with subset deleted=w5265:refnum<vi>[])  [unwired: 1 in]
                n3627 = Insert Into Array(array=w5251, new element #1=w5250, new element #2=w5249, new element #3=w5248, new element #4=w5247, new element #5=w5246, new element #6=w5245) -> (w5244:bool[])  [unwired: 1 in]
                n3628 = Array Subset(array=w5241, index=6 ("索引"), length=2 ("长度")) -> (w5229:bool[])
                n3629 = Array Subset(array=w5238, index=5 ("索引"), length=3 ("长度")) -> (w5230:bool[])
                n3630 = And Array Elements(Boolean array=w5244) -> (logical AND=w5226:bool)
                n3631 = Insert Into Array(array=w5233, new element #1=w5232, new element #2=w5231, new element #3=w5230, new element #4=w5229, new element #5=w5228) -> (w5227:bool[])  [unwired: 1 in]
                n3632 = And Array Elements(Boolean array=w5227) -> (logical AND=w5225:bool)
              }
              frame "单选选项2" {
                n3633 = global read "功能码全局.vi" "18"() -> (w5282:bool[])
                n3634 = global read "功能码全局.vi" "15"() -> (w5303:bool[])
                n3635 = global read "功能码全局.vi" "16"() -> (w5300:bool[])
                n3636 = Delete From Array(array=w5308, index=w5309) -> (deleted portion=w5306:refnum<vi>, array with subset deleted=w5307:refnum<vi>[])  [unwired: 1 in]
                n3637 = Index Array(array=w5300, index #1=4 ("索引"), index #2=5 ("索引"), index #3=6 ("索引"), index #4=7 ("索引")) -> (element #1=w5294:bool, element #2=w5293:bool, element #3=w5289:bool, element #4=w5288:bool)
                n3638 = Index Array(array=w5282, index #1=4 ("索引"), index #2=5 ("索引"), index #3=6 ("索引"), index #4=7 ("索引"), index #5=2 ("索引"), index #6=3 ("索引"), index #7=0 ("索引"), index #8=1 ("索引")) -> (element #1=w5275:bool, element #2=w5278:bool, element #3=w5277:bool, element #4=w5276:bool, element #5=w5274:bool, element #6=w5273:bool, element #7=w5268:bool, element #8=w5269:bool)
                n3639 = Delete From Array(array=w5303, length=4 ("长度"), index=0 ("索引")) -> (deleted portion=w5295:bool[], array with subset deleted=w5290:bool[])
                n3640 = Insert Into Array(array=w5290, new element #1=w5289, new element #2=w5288, new element #3=w5278, new element #4=w5277, new element #5=w5276, new element #6=w5269) -> (w5287:bool[])  [unwired: 1 in]
                n3641 = Insert Into Array(array=w5295, new element #1=w5294, new element #2=w5293, new element #3=w5275, new element #4=w5274, new element #5=w5273, new element #6=w5268) -> (w5292:bool[])  [unwired: 1 in]
                n3642 = And Array Elements(Boolean array=w5292) -> (logical AND=w5291:bool)
                n3643 = And Array Elements(Boolean array=w5287) -> (logical AND=w5286:bool)
              }
            }
            n3644 = property on="全部写入" class="Bool (严格)"("Visible"=w5208) -> ()  [unwired: 2 in, 2 out]
            n3645 = property on="全部读取" class="Bool (严格)"("Visible"=w5207) -> ()  [unwired: 2 in, 2 out]
            n3646 = property on="从板号" class="DigNum (严格)"("Visible"=w5205) -> ()  [unwired: 2 in, 2 out]
            n3647 = local write "主从选择"(w5219) -> ()
            n3648 = property on="从板个数" class="DigNum (严格)"("Visible"=w5211) -> ()  [unwired: 2 in, 2 out]
            n3649 = for {
              tunnel: u32 87470 -> [w5223]
              tunnel: w5216 -> [w5222] mode=indexing
              n3650 = property class="Bool (严格)"(reference=w5222, "BoolText.TextColor"=w5223) -> ()  [unwired: 1 in, 2 out]
            }
            n3651 = Not(x=w5211) -> (.not. x?=w5212:bool)
            n3652 = property class="Bool (严格)"(reference=w5215, "BoolText.TextColor"=u32 16777215) -> ()  [unwired: 1 in, 2 out]
            n3653 = property on="主板选项" class="Tree (严格)"("Visible"=w5211) -> ()  [unwired: 2 in, 2 out]
            n3654 = property on="从板选项" class="Tree (严格)"("Visible"=w5212) -> ()  [unwired: 2 in, 2 out]
            n3655 = property on="当前从板板号" class="DigNum (严格)"("Visible"=w5212) -> ()  [unwired: 2 in, 2 out]
            n3656 = property on="单个读取" class="Bool (严格)"("Visible"=w5206) -> ()  [unwired: 2 in, 2 out]
            n3657 = property on="单个写入" class="Bool (严格)"("Visible"=w5206) -> ()  [unwired: 2 in, 2 out]
          }
          event "从板号": Value Change {
            n3658 = event-data() -> ()  [unwired: 7 out]
            n3659 = local read "key names"() -> (w5311:string[])
            n3660 = Empty Array?(array=w5311) -> (empty?=w5310:bool)
            n3661 = case shown="假" w5310 {
              tunnel: w5311 -> [w5314 _]
              frame False {
                n3662 = stacked-sequence {
                  seq-local: [w5315 _] -> [_ w5378]
                  tunnel: w5314 -> [w5323 _]
                  frame #0 {
                    w5354 = 2 ("长度")
                    w5351 = 20 ("长度")
                    w5339 = 1 ("索引")
                    n3663 = local read "从板号"() -> (w5315:u8)
                    n3664 = local read "输出数组"() -> (w5324:string[][])
                    n3665 = Decrement(x=w5315) -> (x-1=w5321:u8)
                    n3666 = Index Array(array=w5324, index (col)=w5321) -> (element=w5352:string[])  [unwired: 1 in]
                    n3667 = global write "读配置文件全局2.vi" "从板板号"(w5315) -> ()
                    n3668 = Search 1D Array(1D array=w5323, element="风机开启温度" ("元素")) -> (index of element=w5336:i32)  [unwired: 1 in]
                    n3669 = Search 1D Array(1D array=w5323, element="电压过高一级" ("元素"), start index (0)=w5336) -> (index of element=w5334:i32)
                    n3670 = Decrement(x=w5336) -> (x-1=w5338:i32)
                    n3671 = Array Subset(array=w5352, index=w5339, length=w5338) -> (w5322:string[])
                    n3672 = Array Subset(array=w5352, index=w5334, length=21 ("长度")) -> (w5326:string[])
                    n3673 = Array Subset(array=w5323, index=w5339, length=w5338) -> (w5369:string[])
                    n3674 = Array Subset(array=w5352, index=w5336, length=7 ("长度")) -> (w5332:string[])
                    n3675 = for {
                      tunnel: w5326 -> [w5371] mode=indexing
                      tunnel: [w5370] -> w5325 mode=indexing
                      n3676 = Fract/Exp String To Number(string=w5371) -> (number=w5370:dbl)  [unwired: 3 in, 1 out]
                    }
                    n3677 = for {
                      tunnel: w5332 -> [w5373] mode=indexing
                      tunnel: [w5372] -> w5316 mode=indexing
                      n3678 = Fract/Exp String To Number(string=w5373) -> (number=w5372:dbl)  [unwired: 3 in, 1 out]
                    }
                    n3679 = Delete From Array(array=w5325, length=7 ("长度"), index=0 ("索引")) -> (deleted portion=w5319:dbl[], array with subset deleted=w5329:dbl[])
                    n3680 = Array To Cluster(array=w5316) -> (cluster=w5341:T26)
                    n3681 = global write "读配置文件全局2.vi" "加热控制参数"(w5316) -> ()
                    n3682 = Delete From Array(array=w5329, length=7 ("长度"), index=0 ("索引")) -> (deleted portion=w5318:dbl[], array with subset deleted=w5317:dbl[])
                    n3683 = local write "加热控制参数"(w5341) -> ()
                    n3684 = Array To Cluster(array=w5319) -> (cluster=w5366:T26)
                    n3685 = Array To Cluster(array=w5317) -> (cluster=w5368:T26)
                    n3686 = Array To Cluster(array=w5318) -> (cluster=w5367:T26)
                    n3687 = global write "读配置文件全局2.vi" "三级故障阀值"(w5317) -> ()
                    n3688 = global write "读配置文件全局2.vi" "一级故障阀值"(w5319) -> ()
                    n3689 = global write "读配置文件全局2.vi" "二级故障阀值"(w5318) -> ()
                    n3690 = local write "一级故障 6"(w5366) -> ()
                    n3691 = local write "一级故障 8"(w5368) -> ()
                    n3692 = local write "一级故障 7"(w5367) -> ()
                    n3693 = Search 1D Array(1D array=w5369, element="温度个数" ("元素")) -> (index of element=w5348:i32)  [unwired: 1 in]
                    n3694 = Search 1D Array(1D array=w5369, element="第一个保险通道" ("元素")) -> (index of element=w5349:i32)  [unwired: 1 in]
                    n3695 = Search 1D Array(1D array=w5369, element="电压个数" ("元素")) -> (index of element=w5347:i32)  [unwired: 1 in]
                    n3696 = Search 1D Array(1D array=w5369, element="第1通道电压个数" ("元素")) -> (index of element=w5350:i32)  [unwired: 1 in]
                    n3697 = Array Subset(array=w5322, index=w5347, length=2 ("长度")) -> (w5355:string[])
                    n3698 = Array Subset(array=w5322, index=w5348, length=w5354) -> (w5357:string[])
                    n3699 = Array Subset(array=w5322, index=w5349, length=20 ("长度")) -> (w5358:string[])
                    n3700 = Array Subset(array=w5322, index=w5350, length=w5351) -> (w5356:string[])
                    n3701 = Insert Into Array(array=w5355, new element #1=w5356, new element #2=w5357, new element #3=w5358) -> (w5320:string[])  [unwired: 1 in]
                    n3702 = Array Subset(array=w5369, index=w5347, length=w5354) -> (w5359:string[])
                    n3703 = Array Subset(array=w5369, index=w5348, length=w5354) -> (w5361:string[])
                    n3704 = Array Subset(array=w5369, index=w5349, length=w5351) -> (w5362:string[])
                    n3705 = Array Subset(array=w5369, index=w5350, length=w5351) -> (w5360:string[])
                    n3706 = global write "读配置文件全局2.vi" "表格"(w5320) -> ()
                    n3707 = Insert Into Array(array=w5359, new element #1=w5360, new element #2=w5361, new element #3=w5362) -> (w5364:string[])  [unwired: 1 in]
                    n3708 = Build Array(w5364, w5320) -> (w5363:string[][])
                    n3709 = Transpose 2D Array(2D array=w5363) -> (transposed array=w5365:string[][])
                    n3710 = local write "项目信息 2"(w5365) -> ()
                  }
                  frame #1 {
                    n3711 = Number To Decimal String(number=w5378) -> (decimal integer string=w5376:string)  [unwired: 1 in]
                    n3712 = control-ref of="结果"() -> (w5381:refnum<vi>)
                    n3713 = Concatenate Strings("从板", w5376, "导入完成") -> (w5374:string)
                    n3714 = Build Array(w5374) -> (w5379:string[])
                    n3715 = call "表格编辑.vi"("新元素/子数组"=w5379, "活动单元格:单元格背景色"=u32 6618880, "MCListbox引用句柄"=w5381) -> ()  [unwired: 9 out]
                  }
                }
              }
              frame True {
              }
            }
          }
          event "读配置文件": Value Change {
            n3716 = event-data() -> ("NewVal"=w5382:bool)  [unwired: 6 out]
            n3717 = case shown="真" w5382 {
              tunnel: w5386 -> [w5388 w5393]
              tunnel: [w5388 w5392] -> w5385
              tunnel: w5384 -> [w5387 w5391]
              tunnel: [w5387 w5390] -> w5383
              frame False {
              }
              frame True {
                n3718 = Enqueue Element(queue=w5393, element="读配置文件", error in (no error)=w5391) -> (queue out=w5392:refnum<queue>, error out=w5390:errorcluster)  [unwired: 2 out]
                n3719 = call <vilib>:"Set Busy.vi"() -> ()  [unwired: 4 in, 8 out]
              }
            }
          }
          event "保存主板参数": Value Change {
            n3720 = event-data() -> ("NewVal"=w5394:bool)  [unwired: 6 out]
            n3721 = case shown="真" w5394 {
              tunnel: w5398 -> [w5400 w5405]
              tunnel: [w5400 w5404] -> w5397
              tunnel: w5396 -> [w5399 w5403]
              tunnel: [w5399 w5402] -> w5395
              frame False {
              }
              frame True {
                n3722 = Enqueue Element(queue=w5405, element="写配置文件", error in (no error)=w5403) -> (queue out=w5404:refnum<queue>, error out=w5402:errorcluster)  [unwired: 2 out]
              }
            }
          }
          event "继电器全开": Value Change {
            n3723 = event-data() -> ("NewVal"=w5406:bool)  [unwired: 6 out]
            n3724 = case shown="真" w5406 {
              tunnel: w5406 -> [_ w5409]
              frame False {
              }
              frame True {
                n3725 = stacked-sequence {
                  tunnel: w5409 -> [_ w5419 _]
                  frame #0 {
                    w5410 = FALSE ("清BUFF")
                    n3726 = local write "正级继电器"(w5410) -> ()
                    n3727 = local write "负级继电器"(w5410) -> ()
                    n3728 = local write "充电继电器"(w5410) -> ()
                    n3729 = local write "加热继电器"(w5410) -> ()
                    n3730 = local write "风机继电器"(w5410) -> ()
                    n3731 = local write "预充电继电器"(w5410) -> ()
                    n3732 = local write "继电器超时处理"(FALSE ("继电器超时处理")) -> ()
                    n3733 = local write "主从选择"(enum32{"主板", "从板"}."主板" ("主从选择")) -> ()
                    n3734 = local write "清BUFF"(FALSE ("清BUFF")) -> ()
                  }
                  frame #1 {
                    n3735 = case shown="真" w5419 {
                      selector: w5419 -> [_ w5434]
                      frame False {
                      }
                      frame True {
                        w5430 = 256.0 ("y")
                        w5421 = u32 1 ("命令序号")
                        w5420 = u8 192 ("命令")
                        n3736 = local read "动作保持时间"() -> (w5431:dbl)
                        n3737 = Quotient & Remainder(x=w5431, y=w5430) -> (x-y*floor(x/y)=w5423:dbl, floor(x/y)=w5427:dbl)
                        n3738 = Quotient & Remainder(x=w5427, y=w5430) -> (x-y*floor(x/y)=w5424:dbl, floor(x/y)=w5428:dbl)
                        n3739 = Quotient & Remainder(x=w5428, y=w5430) -> (x-y*floor(x/y)=w5425:dbl, floor(x/y)=w5429:dbl)
                        n3740 = local read "设备索引号"() -> (w5438:u16)
                        n3741 = local read "CAN卡类型"() -> (w5439:u32)
                        n3742 = local read "CAN端口"() -> (w5437:u16)
